vi "Detect (ARGB).vi"(5 "Non-Maxium Suppression Threshold":sgl, 7 "Confidence Threshold":sgl=0.5, 8 "error in (no error)":errorcluster, 10 "ARGB Image in":T4, 11 "DNN Detection Model in":refnum<class "DNN Detection Model.lvclass">) -> (0 "error out":errorcluster, 2 "Detections":T1[](array[typedef]), 3 "DNN Detection Model":refnum<class "DNN Detection Model.lvclass">)   [LabVIEW 2020, in "feature_detection.lvlib" / "DNN Detection Model.lvclass"]
uses:
  DNN Detection Model.lvclass
  DNN Detection Model.lvclass/DNN Detection Model.ctl
  e837249a-f575-44a9-ab73-66ed6d7d79a4.vi
  common/Image Point (Float).ctl
  common/common.lvlib
  common/Quad Corners.ctl
  Detection.ctl
  image/ARGB Image.ctl
  image/image.lvlib
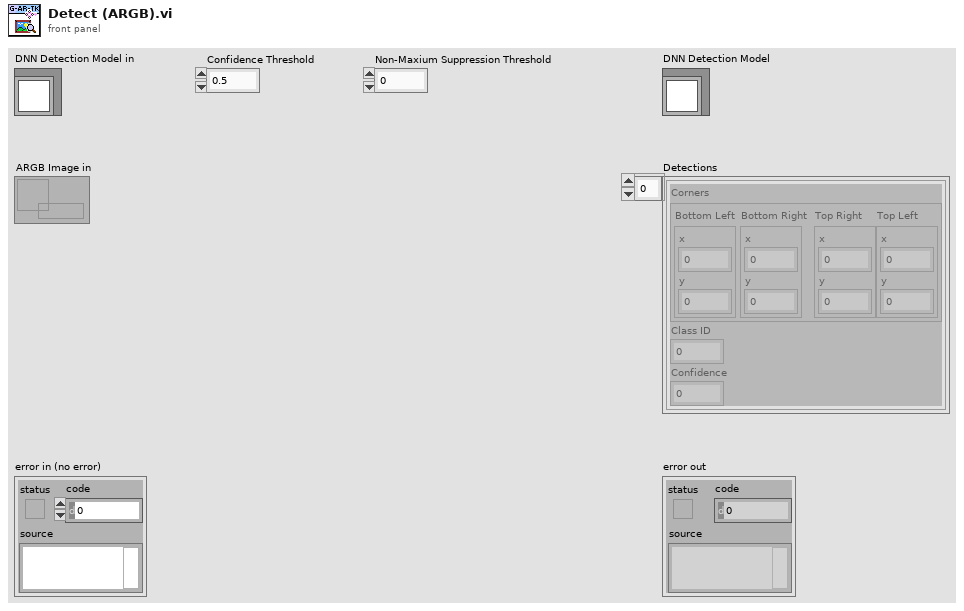
[diagram p1: front panel]
types:
  T1 = typedef "feature_detection.lvlib/DNN Detection Model.lvclass/Detection.ctl" = cluster{"Corners":T2, "Class ID":i32, "Confidence":sgl}
  T2 = typedef "common.lvlib/Quad Corners.ctl" = cluster{"Bottom Left":T3, "Bottom Right":T3, "Top Right":T3, "Top Left":T3}
  T3 = typedef "common.lvlib/Image Point (Float).ctl" = cluster{"x":dbl, "y":dbl}
  T4 = typedef "image.lvlib/ARGB Image.ctl" = refnum<data-value>
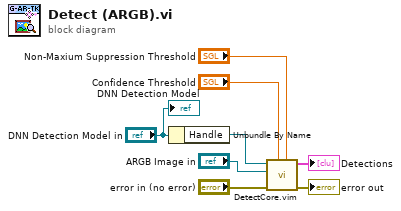
[diagram p0: block diagram]
diagram:
  n1 = Unbundle By Name("DNN Detection Model in") -> ("Handle"=w5:refnum<data-value>)
  n2 = call "DetectCore.vim"("Non-Maxium Suppression Threshold"="Non-Maxium Suppression Threshold", "Confidence Threshold"="Confidence Threshold", "error in (no error)"="error in (no error)", "Image in"="ARGB Image in", "Detection Model"=w5) -> ("error out"=→"error out":errorcluster, "Detections"=→"Detections":T1[])  [unwired: 5 in]
  "DNN Detection Model" <- "DNN Detection Model in"
